vi "drawPicbyArr.vi"(11 "Array":u8[][](array[numeric])) -> (3 "2D Picture":picture)   [LabVIEW 2024]
panel:
  in  "color map":u32[](array[colorbox])
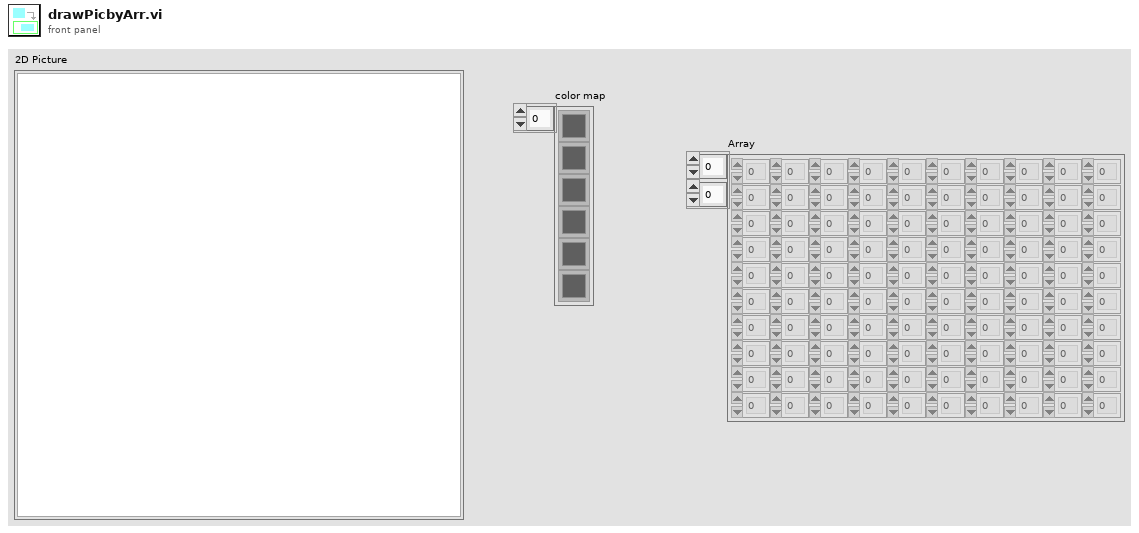
[diagram p1: front panel]
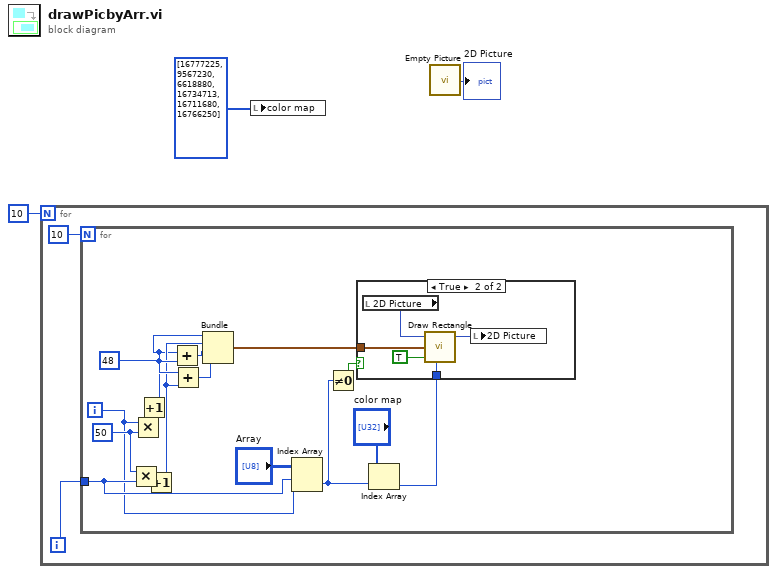
[diagram p0: block diagram]
diagram:
  n1 = for {
    N: 10 -> [_]
    i -> [w4]
    n2 = for {
      N: 10 -> [_]
      tunnel: w4 -> [w13]
      i -> [w12]
      w19 = 48 ("y")
      w14 = 50 ("y")
      n3 = Multiply(x=w14, y=w13) -> (x*y=w15:i32)
      n4 = Multiply(x=w12, y=w14) -> (x*y=w21:i32)
      n5 = Increment(x=w21) -> (x+1=w8:i32)
      n6 = Increment(x=w15) -> (x+1=w9:i32)
      n7 = Add(x=w8, y=w19) -> (x+y=w20:i32)
      n8 = Add(x=w19, y=w9) -> (x+y=w18:i32)
      n9 = Bundle(w8, w9, w20, w18) -> (w17:cluster{i32, i32, i32, i32})  [unwired: 1 in]
      n10 = Index Array(array="Array", index (row)=w13, index (col)=w12) -> (element=w7:u8)
      n11 = Not Equal To 0?(x=w7) -> (x != 0?=w6:bool)
      n12 = Index Array(array="color map", index=w7) -> (element=w10:u32)
      n13 = case shown="True" w6 {
        tunnel: w17 -> [_ w24]
        tunnel: w10 -> [_ w22]
        frame False {
        }
        frame True {
          n14 = local read "2D Picture"() -> (w25:picture)
          n15 = call <vilib>:"Draw Rectangle.vi"("picture"=w25, "rect"=w24, "fill?(F)"=TRUE, "color(black)"=w22) -> ("new picture"=w23:picture)  [unwired: 5 in]
          n16 = local write "2D Picture"(w23) -> ()
        }
      }
    }
  }
  n17 = local write "color map"(u32[] [16777225, 9567230, 6618880, 16734713, 16711680, 16766250]) -> ()
  n18 = call "Empty Picture"() -> ("empty picture"=→"2D Picture":picture)
